vi "HEWH Remaining Time.vi"(9 "Ideal Purge Time":dbl, 10 "Current Draw Timer":dbl, 11 "Total Test Timer (1hr)":dbl) -> (1 "Purge Time":dbl, 2 "Start Draw/Purge Sequence":bool, 3 "Test Complete":bool)   [LabVIEW 2019]
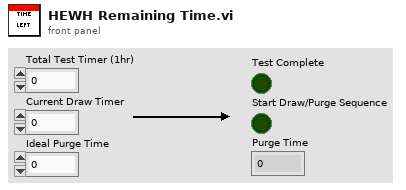
[diagram p1: front panel]
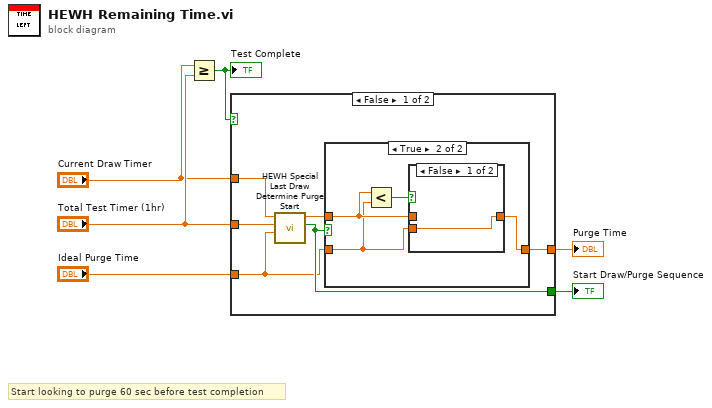
[diagram p0: block diagram]
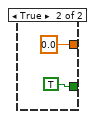
[diagram p4: hidden frame]
diagram:
  # "Start looking to purge 60 sec before test completion"
  n1 = Greater Or Equal?(x="Current Draw Timer", y="Total Test Timer (1hr)") -> (x >= y?=w3:bool)
  "Test Complete" <- w3
  n2 = case shown="False" w3 {
    tunnel: "Total Test Timer (1hr)" -> [w7 _]
    tunnel: "Current Draw Timer" -> [w8 _]
    tunnel: [w12 TRUE] -> w6
    tunnel: "Ideal Purge Time" -> [w11 _]
    tunnel: [w10 0.0 ("Ideal Purge Time")] -> w4
    frame False {
      n3 = call "HEWH Special Last Draw Determine Purge Start.vi"("Ideal Purge Time"=w11, "Total Test Timer (1hr)"=w7, "Current Draw Timer"=w8) -> ("Start Purge"=w12:bool, "Seconds Until EOT"=w9:dbl)  [unwired: 6 in, 1 out]
      n4 = case shown="True" w12 {
        tunnel: w9 -> [_ w16]
        tunnel: w11 -> [w13 w14]
        tunnel: [w13 w15] -> w10
        frame False {
        }
        frame True {
          n5 = Less?(x=w16, y=w14) -> (x < y?=w17:bool)
          n6 = case shown="False" w17 {
            tunnel: [w18 w19] -> w15
            tunnel: w16 -> [_ w19]
            tunnel: w14 -> [w18 _]
            frame False {
            }
            frame True {
            }
          }
        }
      }
    }
    frame True {
    }
  }
  "Start Draw/Purge Sequence" <- w6
  "Purge Time" <- w4
